vi "sensor-csv-to-data.vi"(9 "no. datapoints":i32, 11 "sensor-name":string) -> (0 "data output":T1 {"Humidity (%)" format="%.2f"; "Temp (degC)" format="%.2f"; "CO2 (ppm)" format="%.2f"}, 1 "SCD41: Humidity (%)":dbl format="%.2f", 2 "SCD41: Temp (degC)":dbl format="%.2f", 3 "SCD41: CO2 (ppm)":dbl format="%.2f")   [LabVIEW 2021]
uses:
  SCD41.ctl
  <vilib>/regexp/Match Regular Expression.xnode
panel:
  in  "sensor-type":string
  in  "sensor-csv-input":string
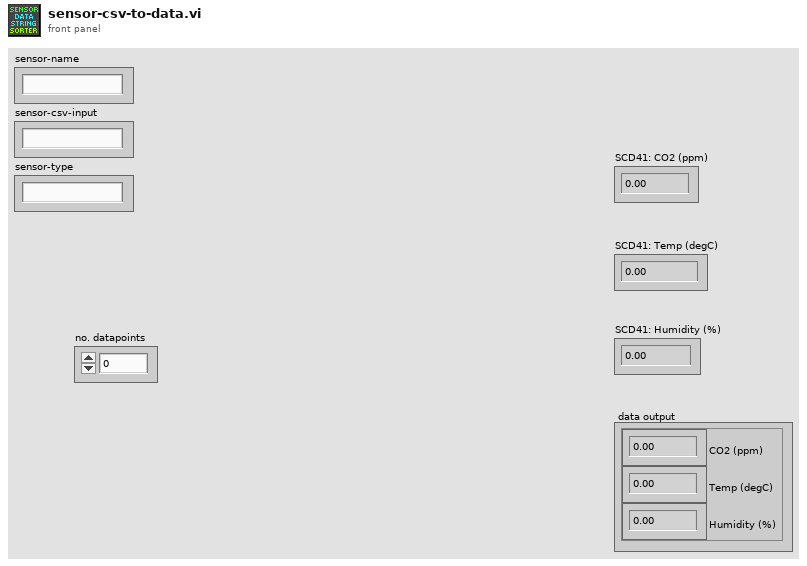
[diagram p1: front panel]
types:
  T1 = typedef "SCD41.ctl" = cluster{"CO2 (ppm)":dbl, "Temp (degC)":dbl, "Humidity (%)":dbl}
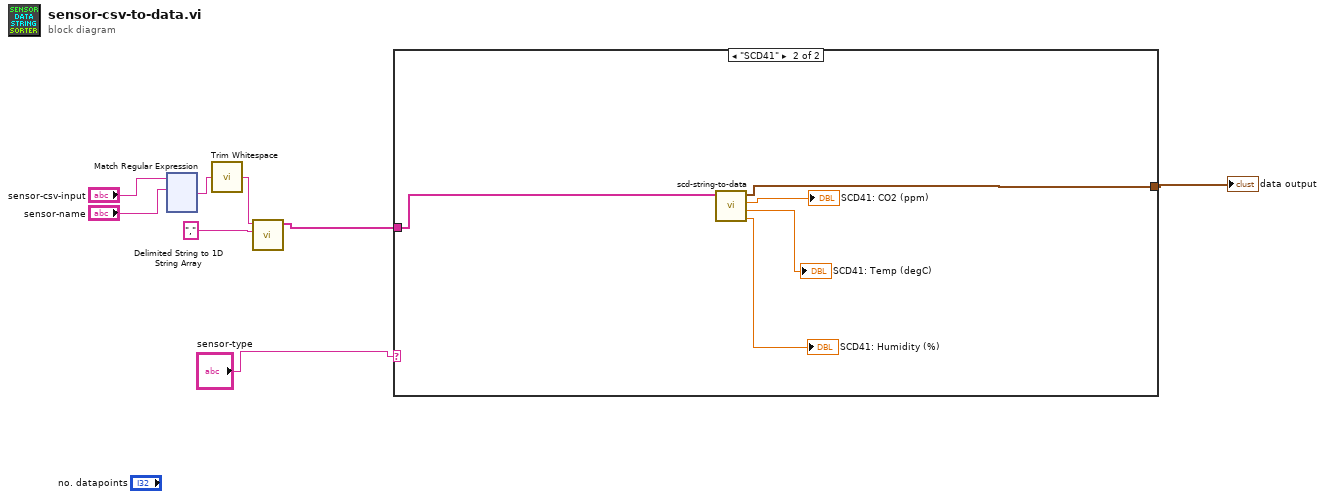
[diagram p0: block diagram]
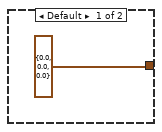
[diagram p2: hidden frame]
diagram:
  n1 = xnode "Match Regular Expression"("input string"="sensor-csv-input", "regular expression"="sensor-name") -> ("after match"=w6:string)  [unwired: 4 in, 4 out]
  n2 = call <vilib>:"Trim Whitespace.vi"("string"=w6) -> ("trimmed string"=w8:string)  [unwired: 1 in]
  n3 = call <vilib>:"Delimited String to 1D String Array.vi"("delimiter"=",", "delimited string"=w8) -> ("string array"=w3:string[])  [unwired: 9 in]
  n4 = case shown="\"SCD41\"" "sensor-type" {
    tunnel: w3 -> [_ w14]
    tunnel: [T1 {"CO2 (ppm)"=0.0, "Temp (degC)"=0.0, "Humidity (%)"=0.0} ("SCD typedef") w12] -> w2
    frame Default {
    }
    frame "SCD41" {
      n5 = call "scd-string-to-data.vi"("string input"=w14) -> ("SCD41: Humidity (%)"=→"SCD41: Humidity (%)":dbl, "SCD41: Temp (degC)"=→"SCD41: Temp (degC)":dbl, "SCD41: CO2 (ppm)"=→"SCD41: CO2 (ppm)":dbl, "SCD typedef"=w12:T1)  [unwired: 7 in]
    }
  }
  "data output" <- w2
